vi "Safe Shooter Mode.vi"(10 "Ball Detected?":bool, 11 "Shooter Commands":T2={"Command"=enum."Prime Shooter", "Mode"=enum."Manual", "Shot Type"=enum."Batter Shot", "Override Trigger IR"=FALSE}) -> (1 "Trigger Power":dbl, 2 "Right Power":dbl, 3 "Left Power":dbl, 4 "RPM Ready?":bool, 5 "State":T1, 6 "Shooter Ready?":bool, 7 "Vision Ready?":bool)   [LabVIEW 2015]
uses:
  Common Code/Shooter Command Cluster.ctl
  Common Code/Shooter Commands.ctl
  Common Code/Shoot Modes Enum.ctl
  Common Code/Shot Type.ctl
  Common Code/Shooter State.ctl
  Common Code/Change Detect Int.vi
  Common Code/Change Detect Boolean.vi
  Robot Global Data.vi
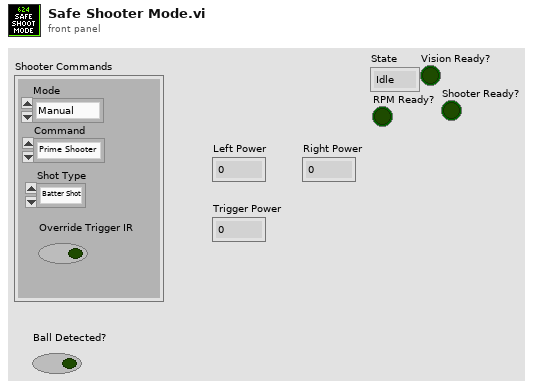
[diagram p1: front panel]
types:
  T1 = typedef "Shooter State.ctl" = enum16{"Idle", "Warmup", "Shooter Ready", "Shoot"}
  T2 = typedef "Shooter Command Cluster.ctl" = cluster{"Command":T3, "Mode":T4, "Shot Type":T5, "Override Trigger IR":bool}
  T3 = typedef "Shooter Commands.ctl" = enum16{"Idle", "Prime Shooter", "Shoot"}
  T4 = typedef "Shoot Modes Enum.ctl" = enum16{"Manual", "Safe", "Auto"}
  T5 = typedef "Shot Type.ctl" = enum16{"Batter Shot", "Curve Shot", "Vision Shot", "Deep Middle Shot"}
  T6 = typedef "Drivetrain Status Cluster.ctl" = cluster{"Modes":T7, "Y (Throttle)":dbl, "X (Steer)":dbl, "Gyro In Range?":bool, "Distance Drive Finished?":bool, "Stop Eject Lockout":bool, "Dist Drive Status":T8, "Y Target":dbl, "Heading Target":dbl, "Vision Target Aligned?":bool, "Gear":dbl, "1st Gear Time":dbl, "2nd Gear Time":dbl, "1st Gear Shifts":dbl, "2nd Gear Shifts":dbl}
  T7 = typedef "Drivetrain Modes.ctl" = enum16{"Climb", "Manual", "Ball Vision Targeting", "Goal Vision Targeting", "PID Distance Drive", "Hybrid"}
  T8 = typedef "Dist Drive Status.ctl" = cluster{"Y In Range":bool, "X In Range":bool, "Gyro In Range":bool, "Y Dist":dbl, "X Dist":dbl, "Gyro":dbl}
  T9 = typedef "Dashboard Control Data.ctl" = cluster{"Shooter Presets":T10, "Encoder Control":T12, "Steer PID output":cluster{"output high":dbl, "output low":dbl}, " Steer PID gains":cluster{"proportional gain (Kc)":dbl, "integral time (Ti, min)":dbl, "derivative time (Td, min)":dbl}, "Drivetrain Settings":T13, "Vision Packet":T14, "Dashboard Drivetrain Command":T15, "Info/Command Cluster":T17, "Ball Vision Packet":T18, "Intake Presets":T20}
  T10 = typedef "Shooter Presets.ctl" = cluster{"Batter Shot":T11, "Low Bar Curve Shot":T11, "Deep Middle Shot":T11, "Manual Shot":T11, "Left Ticks Per Rotation":dbl, "Right Ticks Per Rotation":dbl, "Low Bar Shot":T11, "Shooter RPM Tolerance":dbl, "IIR Filter Power":dbl, "Trigger Power":dbl, "Fire from Load Delay":i32, "Angle Pot Scale Factor":dbl, "Angle Pot Zero":dbl, "Shooter Deck Length":dbl, "String Pot Dist From Pivot":dbl, "Angle PID gains":cluster{"proportional gain (Kc)":dbl, "integral time (Ti, min)":dbl, "derivative time (Td, min)":dbl}, "Angle Motor Output Range":cluster{"output high":dbl, "output low":dbl}, "Shooter Angle Tolerance":dbl, "Vision Shoot m":dbl, "Vision Shoot b":dbl, "Dist from Axis Cam to Pivot":dbl, "High Goal Center Height":dbl, "Feed Forward Max Accel":dbl, "Feed Forward Kv":dbl, "Backwards Trigger":dbl, "Shot Finish Delay (ms)":dbl, "Angle Max Current":dbl, "Angle Current Trip Time":dbl}
  T11 = typedef "Shot Presets.ctl" = cluster{"Left Wheel RPM":dbl, "Right Wheel RPM":dbl, "Angle":dbl}
  T12 = typedef "Encoder Control.ctl" = cluster{"Right Tick Constant":dbl, "Left Tick Constant":dbl, "Reset?":bool, "Y Dist":cluster{"PID gains":cluster{"proportional gain (Kc)":dbl, "integral time (Ti, min)":dbl, "derivative time (Td, min)":dbl}}, "Y Stop Thresh":dbl, "Y Stop Speed":dbl}
  T13 = typedef "Drivetrain Settings.ctl" = cluster{"Gyro Tolerance":dbl, "Throttle Ramp (ms)":dbl, "Angular rate compensation":bool, "Throttle to Rate Scale":dbl, "Rate compensation gain":dbl, "Kv":dbl, "Ka":dbl, "Feed Forward P":dbl, "Feed Forward D":dbl}
  T14 = typedef "Goal Vision Packet.ctl" = cluster{"Distance":dbl, "Center X":dbl, "Center Y":dbl, "Found Target?":bool}
  T15 = typedef "Dashboard Drivetrain Command.ctl" = cluster{"Drivetrain Vision":T16, "Vision Scale Down Speed":dbl, "Vision PID gains":cluster{"proportional gain (Kc)":dbl, "integral time (Ti, min)":dbl, "derivative time (Td, min)":dbl}}
  T16 = typedef "Drivetrain Vision.ctl" = cluster{"High parameters":dbl, "Low parameters":dbl}
  T17 = typedef "Ball Tracking Command Cluster.ctl" = cluster{"Distance to Ball":dbl, "Desired Angle":dbl, "Command":enum16{"Turn to Ball", "Turn to Angle", "Get Distance"}, "Pixels from Center":dbl}
  T18 = typedef "Ball Vision Packet.ctl" = cluster{"Ball Detected?":bool, "Distance to Ball":dbl, "Desired Angle":dbl, "Pixels from Center":dbl, "Tracking mode":T19}
  T19 = typedef "Tracking Mode.ctl" = enum16{"Turn to Ball", "Turn to Angle"}
  T20 = typedef "Intake Presets.ctl" = cluster{"Intake Speed":dbl, "Outake Speed":dbl, "Low Height":dbl, "High Height":dbl, "Full Height":dbl, "Angle Speed":dbl, "Fast Angle":dbl, "Encoder Scale Factor":dbl, "Load Height":dbl, "Output Range":T21, "PID Params":cluster{"PID gains":cluster{"proportional gain (Kc)":dbl, "integral time (Ti, min)":dbl, "derivative time (Td, min)":dbl}}, "Rotation Power Max/Min":dbl}
  T21 = typedef "Drivetrain Output Range.ctl" = cluster{"output high":dbl, "output low":dbl}
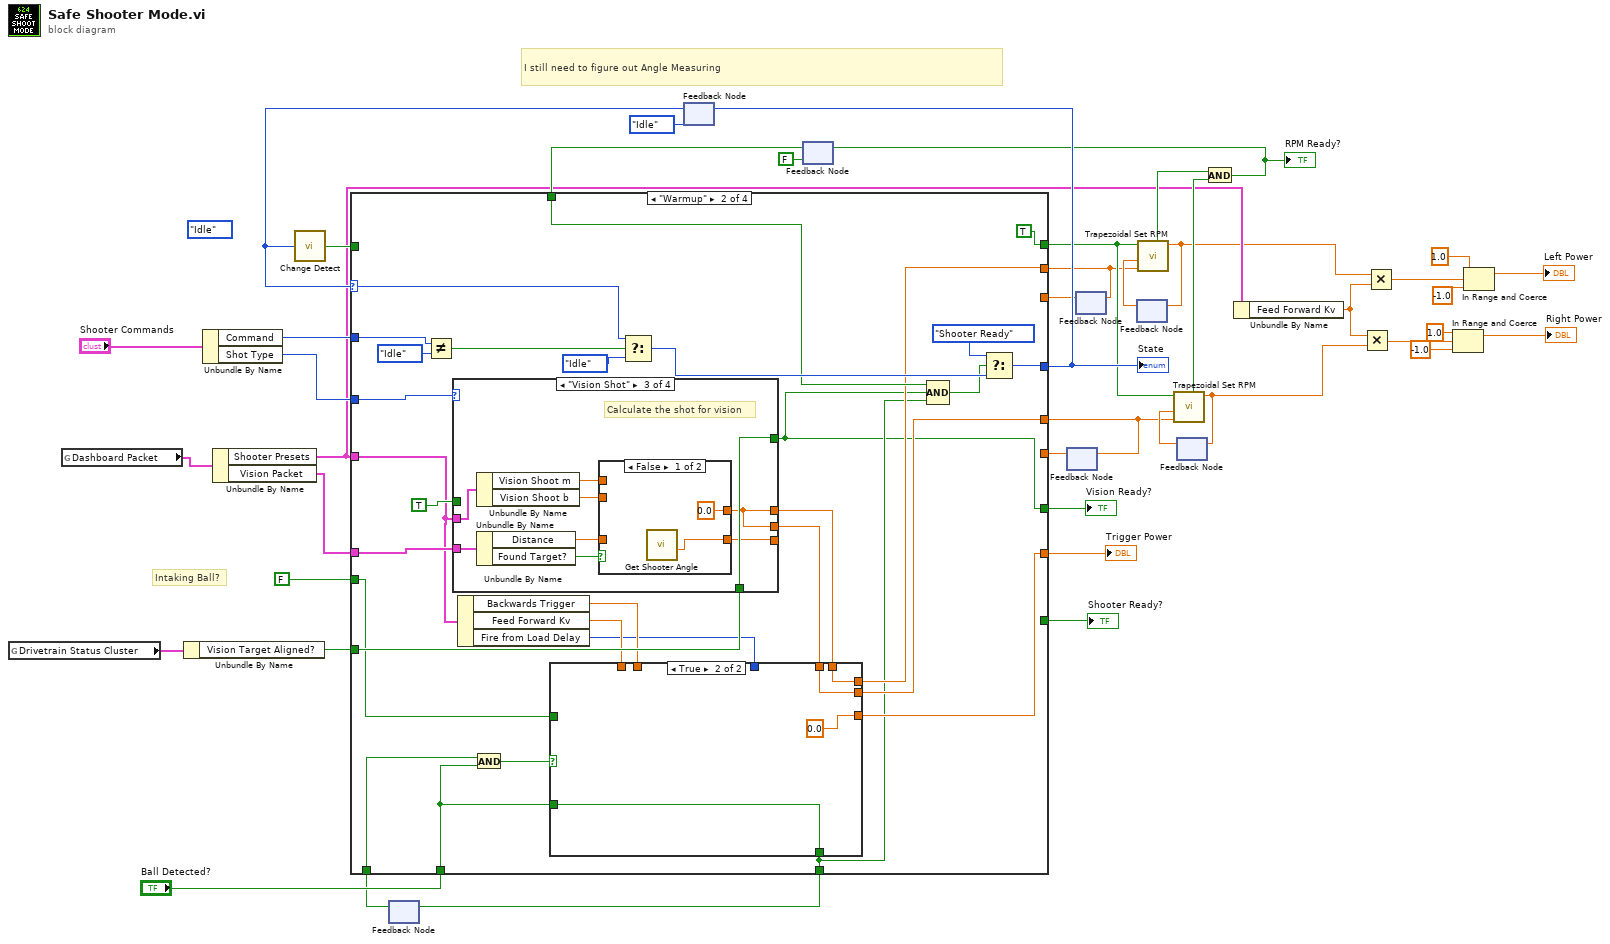
[diagram p0: block diagram]
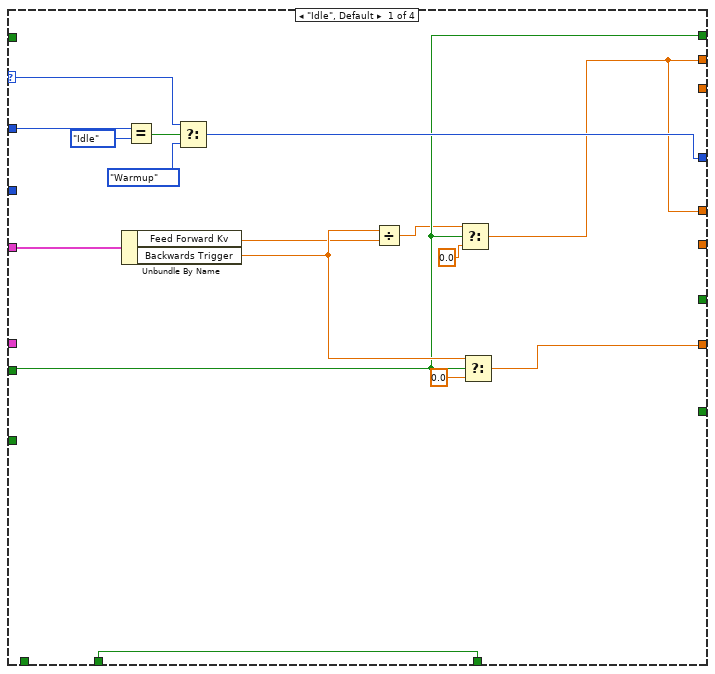
[diagram p2: hidden frame]
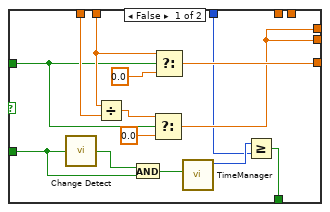
[diagram p3: hidden frame]
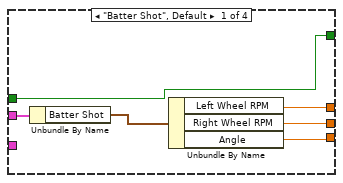
[diagram p4: hidden frame]
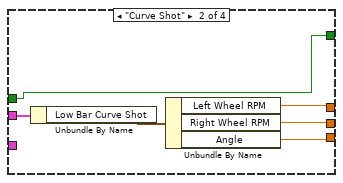
[diagram p5: hidden frame]
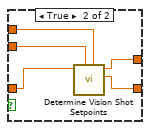
[diagram p6: hidden frame]
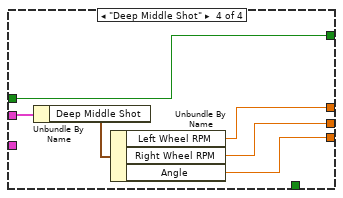
[diagram p7: hidden frame]
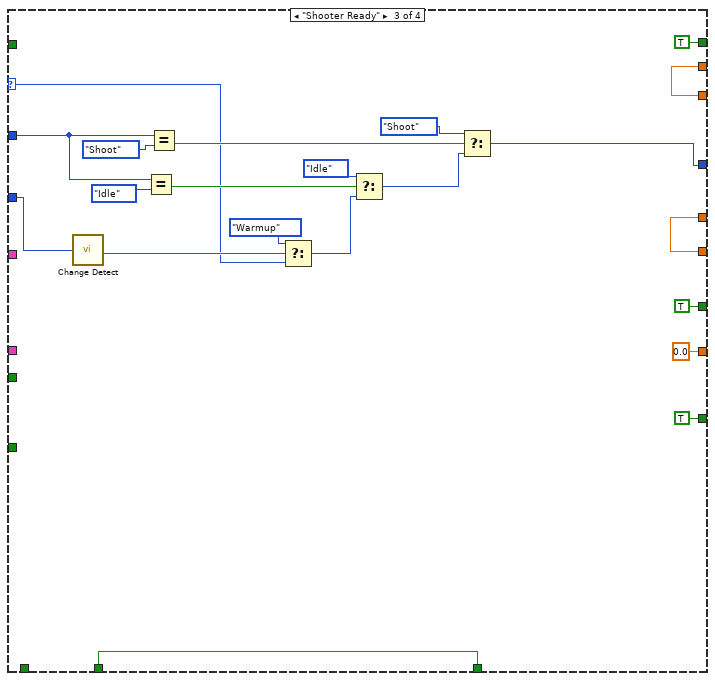
[diagram p8: hidden frame]
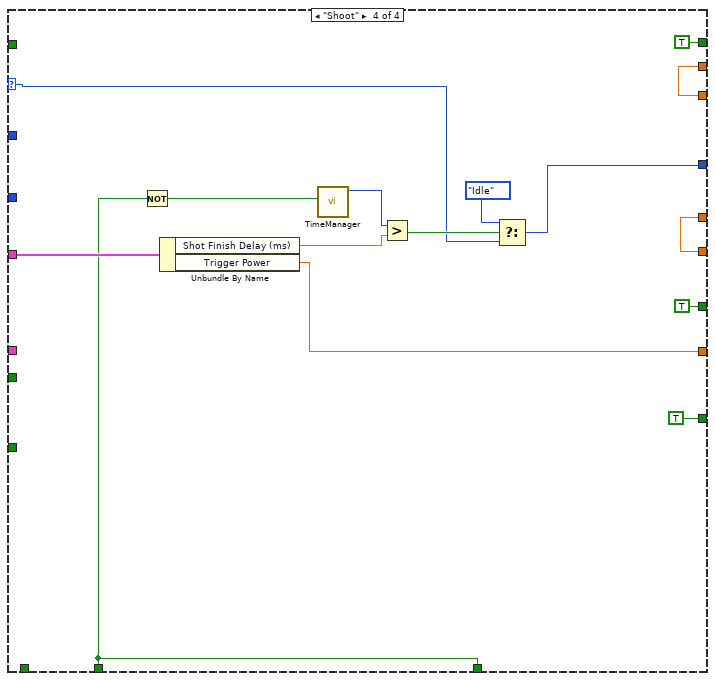
[diagram p9: hidden frame]
diagram:
  (unwired) Shooter_Commands."Idle" ("Command")
  # "I still need to figure out Angle Measuring"
  # "Intaking Ball?"
  n1 = global read "Robot Global Data.vi" "Drivetrain Status Cluster"() -> (w30:T6)
  n2 = global read "Robot Global Data.vi" "Dashboard Packet"() -> (w32:T9)
  n3 = Unbundle By Name(w30) -> ("Vision Target Aligned?"=w29:bool)
  n4 = Unbundle By Name("Shooter Commands") -> ("Command"=w36:T3, "Shot Type"=w33:T5)
  n5 = Unbundle By Name(w32) -> ("Shooter Presets"=w14:T10, "Vision Packet"=w31:T14)
  n6 = feedback #1() -> (w16:bool)  [unwired: 1 in]
  n7 = feedback #2(Shooter_State."Idle" ("Enum")) -> (w35:T1)
  n8 = call-poly "Change Detect.vi"("In"=w35) -> ("Changed?"=w34:bool)
  n9 = feedback #3(FALSE ("Shooter Ready?")) -> (w39:bool)
  n10 = feedback #4() -> (w22:dbl)  [unwired: 1 in]
  n11 = feedback #5() -> (w20:dbl)  [unwired: 1 in]
  n12 = case shown="\"Warmup\"" w35 {
    selector: w35 -> [w55 w84 w150 w167]
    tunnel: [w46 TRUE TRUE TRUE] -> w28
    tunnel: [w44 w69 w160 w175] -> w21
    tunnel: w39 -> [_ w75 _ _]
    tunnel: [w53 w80 w145 w165] -> w37
    tunnel: w36 -> [w58 w87 w155 _]
    tunnel: w34 -> [_ _ _ _]
    tunnel: w33 -> [_ w79 w152 _]
    tunnel: w14 -> [w52 w65 _ w173]
    tunnel: w31 -> [_ w78 _ _]
    tunnel: w29 -> [_ w76 _ _]
    tunnel: [w44 w68 w161 w174] -> w23
    tunnel: w22 -> [_ _ w161 w174]
    tunnel: w20 -> [_ _ w160 w175]
    tunnel: "Ball Detected?" -> [w43 w61 w143 w164]
    tunnel: [w50 w67 0.0 ("Trigger Power") w172] -> w19
    tunnel: FALSE -> [w46 w66 _ _]
    tunnel: w16 -> [_ w73 _ _]
    tunnel: [w43 w60 w143 w164] -> w15
    tunnel: [_ w59 TRUE ("Vision Target Aligned?") TRUE ("Vision Target Aligned?")] -> w2
    tunnel: [_ _ TRUE ("Vision Target Aligned?") TRUE ("Vision Target Aligned?")] -> w1
    frame "Idle", Default {
      n13 = Unbundle By Name(w52) -> ("Feed Forward Kv"=w48:dbl, "Backwards Trigger"=w49:dbl)
      n14 = Equal?(x=w58, y=Shooter_Commands."Idle") -> (x = y?=w56:bool)
      n15 = Select(t=w55, s=w56, f=Shooter_State."Warmup") -> (s? t:f=w53:T1)
      n16 = Divide(x=w49, y=w48) -> (x/y=w45:dbl)
      n17 = Select(t=w45, s=w46, f=0.0) -> (s? t:f=w44:dbl)
      n18 = Select(t=w49, s=w46, f=0.0) -> (s? t:f=w50:dbl)
    }
    frame "Warmup" {
      n19 = Not Equal?(x=w87, y=Shooter_Commands."Idle") -> (x != y?=w85:bool)
      n20 = case shown="\"Vision Shot\"" w79 {
        tunnel: w65 -> [w112 w118 w126 w140]
        tunnel: [w110 w116 w121 w138] -> w70
        tunnel: [w109 w115 w121 w137] -> w71
        tunnel: w78 -> [_ _ w123 _]
        tunnel: [w108 w114 w127 w136] -> w59
        tunnel: w76 -> [_ _ w127 _]
        tunnel: TRUE -> [w108 w114 _ w136]
        tunnel: [w107 w113 w122 w135] -> _
        frame "Batter Shot", Default {
          n21 = Unbundle By Name(w112) -> ("Batter Shot"=w111:T11)
          n22 = Unbundle By Name(w111) -> ("Left Wheel RPM"=w110:dbl, "Right Wheel RPM"=w109:dbl, "Angle"=w107:dbl)
        }
        frame "Curve Shot" {
          n23 = Unbundle By Name(w118) -> ("Low Bar Curve Shot"=w117:T11)
          n24 = Unbundle By Name(w117) -> ("Left Wheel RPM"=w116:dbl, "Right Wheel RPM"=w115:dbl, "Angle"=w113:dbl)
        }
        frame "Vision Shot" {
          # "Calculate the shot for vision"
          n25 = Unbundle By Name(w126) -> ("Vision Shoot m"=w119:dbl, "Vision Shoot b"=w120:dbl)
          n26 = Unbundle By Name(w123) -> ("Distance"=w125:dbl, "Found Target?"=w124:bool)
          n27 = case shown="False" w124 {
            tunnel: w125 -> [_ w134]
            tunnel: [w128 w133] -> w122
            tunnel: [0.0 ("Power") w132] -> w121
            tunnel: w120 -> [_ w131]
            tunnel: w119 -> [_ w130]
            frame False {
              n28 = call "Get Shooter Angle.vi"() -> ("Current Angle"=w128:dbl)  [unwired: 11 in]
            }
            frame True {
              n29 = call "Determine Vision Shot Setpoints.vi"("M"=w130, "B"=w131, "Distance from Target"=w134) -> ("Angle"=w133:dbl, "RPM Power"=w132:dbl)  [unwired: 7 in]
            }
          }
        }
        frame "Deep Middle Shot" {
          n30 = Unbundle By Name(w140) -> ("Deep Middle Shot"=w139:T11)
          n31 = Unbundle By Name(w139) -> ("Left Wheel RPM"=w138:dbl, "Right Wheel RPM"=w137:dbl, "Angle"=w135:dbl)
        }
      }
      n32 = Unbundle By Name(w65) -> ("Backwards Trigger"=w64:dbl, "Feed Forward Kv"=w63:dbl, "Fire from Load Delay"=w62:i32)
      n33 = And(x=w73, y=w61) -> (x .and. y?=w72:bool)
      n34 = case shown="True" w72 {
        tunnel: w71 -> [_ w105]
        tunnel: w70 -> [_ w106]
        tunnel: [w95 w106] -> w69
        tunnel: [w95 w105] -> w68
        tunnel: [w101 0.0 ("Trigger Power")] -> w67
        tunnel: w66 -> [w97 _]
        tunnel: w64 -> [w100 _]
        tunnel: w63 -> [w99 _]
        tunnel: w62 -> [w90 _]
        tunnel: w61 -> [w91 w103]
        tunnel: [w89 w103] -> w60
        frame False {
          n35 = call-poly "Change Detect.vi"("In"=w91) -> ("Changed?"=w94:bool)
          n36 = Divide(x=w100, y=w99) -> (x/y=w98:dbl)
          n37 = And(x=w94, y=w91) -> (x .and. y?=w93:bool)
          n38 = Select(t=w98, s=w97, f=0.0) -> (s? t:f=w95:dbl)
          n39 = Select(t=w100, s=w97, f=0.0) -> (s? t:f=w101:dbl)
          n40 = call "TimeManager.vi"("Reset?"=w93) -> ("Time Since Reset"=w92:u32)  [unwired: 9 in, 1 out]
          n41 = Greater Or Equal?(x=w92, y=w90) -> (x >= y?=w89:bool)
        }
        frame True {
        }
      }
      n42 = Select(t=w84, s=w85, f=Shooter_State."Idle") -> (s? t:f=w83:T1)
      n43 = Compound Arithmetic op=AND(w75, w59, w60) -> (w74:bool)
      n44 = Select(t=Shooter_State."Shooter Ready", s=w74, f=w83) -> (s? t:f=w80:T1)
    }
    frame "Shooter Ready" {
      n45 = call-poly "Change Detect.vi"("In"=w152) -> ("Changed?"=w151:bool)
      n46 = Equal?(x=w155, y=Shooter_Commands."Idle") -> (x = y?=w154:bool)
      n47 = Equal?(x=w155, y=Shooter_Commands."Shoot") -> (x = y?=w158:bool)
      n48 = Select(t=Shooter_State."Warmup", s=w151, f=w150) -> (s? t:f=w148:T1)
      n49 = Select(t=Shooter_State."Idle", s=w154, f=w148) -> (s? t:f=w147:T1)
      n50 = Select(t=Shooter_State."Shoot", s=w158, f=w147) -> (s? t:f=w145:T1)
    }
    frame "Shoot" {
      n51 = Not(x=w164) -> (.not. x?=w171:bool)
      n52 = Unbundle By Name(w173) -> ("Shot Finish Delay (ms)"=w169:dbl, "Trigger Power"=w172:dbl)
      n53 = call "TimeManager.vi"("Reset?"=w171) -> ("Time Since Reset"=w170:u32)  [unwired: 9 in, 1 out]
      n54 = Greater?(x=w170, y=w169) -> (0:w168:bool)
      n55 = Select(t=Shooter_State."Idle", s=w168, f=w167) -> (s? t:f=w165:T1)
    }
  }
  "Trigger Power" <- w19
  "State" <- w37
  "Vision Ready?" <- w2
  "Shooter Ready?" <- w1
  n56 = feedback-in #1(w15) -> ()
  n57 = feedback-in #2(w37) -> ()
  n58 = feedback-in #4(w23) -> ()
  n59 = feedback-in #5(w21) -> ()
  n60 = feedback #6() -> (w40:dbl)  [unwired: 1 in]
  n61 = call "Trapezoidal Set RPM.vi"("Desired RPM"=w21, "Current RPM"=w40, "Spinning Wheels?"=w28) -> ("RPM"=w11:dbl, "Shooter Ready?"=w26:bool)  [unwired: 6 in, 1 out]
  n62 = feedback-in #6(w11) -> ()
  n63 = feedback #7() -> (w24:dbl)  [unwired: 1 in]
  n64 = call "Trapezoidal Set RPM.vi"("Desired RPM"=w23, "Current RPM"=w24, "Spinning Wheels?"=w28) -> ("RPM"=w12:dbl, "Shooter Ready?"=w27:bool)  [unwired: 6 in, 1 out]
  n65 = feedback-in #7(w12) -> ()
  n66 = And(x=w26, y=w27) -> (x .and. y?=w25:bool)
  "RPM Ready?" <- w25
  n67 = feedback-in #3(w25) -> ()
  n68 = Unbundle By Name(w14) -> ("Feed Forward Kv"=w13:dbl)
  n69 = Multiply(x=w13, y=w12) -> (x*y=w10:dbl)
  n70 = Multiply(x=w11, y=w13) -> (x*y=w4:dbl)
  n71 = In Range and Coerce(upper limit=1.0, x=w10, lower limit=-1.0) -> (coerced(x)=→"Right Power":dbl)  [unwired: 1 out]
  n72 = In Range and Coerce(upper limit=1.0, x=w4, lower limit=-1.0) -> (coerced(x)=→"Left Power":dbl)  [unwired: 1 out]
